vi "sych2SQL.vi"(11 "Data\\":path=path "\\\\192.168.1.45\\du lieu kho/data") -> ()   [LabVIEW 2015]
uses:
  <vilib>/addons/database/Connection.llb/Conn ObjectReference.ctl
  <vilib>/Utility/miscctls.llb/LVRowAndColumnUnsignedTypeDef.ctl
  <vilib>/addons/database/Connection.llb/DB Tools Open Connec (String).vi
  <vilib>/addons/database/Connection.llb/Conn Execute.vi
  <vilib>/addons/database/Recordset.llb/Rec Destroy - Connection.vi
  <vilib>/addons/database/NI_Database_API.lvlib
panel:
  out "error out 9":errorcluster
  out "Numeric 2":i32
  out "error out 8":errorcluster
  out "error out 3":errorcluster
  out "Array":errorcluster[](array[cluster])
  in  "connection reference 3":T1
  in  "connection reference 2":T1
  out "Numeric":i32
  out "error out 7":errorcluster
  out "error out 6":errorcluster
  out "error out 5":errorcluster
  out "error out 4":errorcluster
  out "error out 2":errorcluster
  out "error out":errorcluster
  in  "Lot Size":dbl
  out "Table 2":string[][](table)
  in  "Amount (F4)":dbl caption="(F4)"
  in  "Item Code (F3)":string
  out "ECODE":string
  in  "Input Date":timestamp format="%<%d/%m/%Y>T"
  out "Input No.":string
  in  "Product":string(combo)
  in  "Quantity":dbl
  in  "Location":string
  in  "Maker":string(combo)
  in  "Lot Maker":string
  in  "Maker Code":string
  in  "Unit 2":string
  in  "AUTO_PRINT":bool caption="AUTO"
  in  "connection reference":T1
  out "password":cluster{"ID":string, "Password":string}[](array[cluster])
  in  "Next Button 2":bool
  in  "Find":string
  out "Find Array":i32[](array[numeric])
  in  "output cluster 2":cluster{"ID":string, "Password":string}
  out "Worker Code":string
  out "record(s) 3":T2(array[cluster])
  in  "element 3":T3
  in  "Ring":u16(ring) items=["INVOICE", "LINE"]
  in  "element":T3
  out "record(s)":T2(array[cluster])
  in  "End":bool
  out "Item code":string[](array[string])
  out "Item data":T4(array[cluster])
  out "Initial":i32
  out "Output":i32
  out "Input":i32
  in  "Initial Date":string
  in  "Item type":T5
  in  "DATE":string
  in  "Invoice Date":string
  in  "Exit":bool
  in  "output array":string[][](array[string])=[["", "", "", "", "", "", "", ""]]
  in  "PRODUCT":string
  in  "input array":string[][](array[string])=[["", "", "", "", "", "", "", ""]]
  in  "Check":bool
  in  "Table":string[][](table)=[["", "", "", "", "", "", "", ""], ["", "", "", "", "", "", "", ""], ["", "", "", "", "", "", "", ""], ["", "", "", "", "", "", "", ""], ["", "", "", "", "", "", "", ""], ["", "", "", "", "", "", "", ""]]
  # "CHECK STOCK"
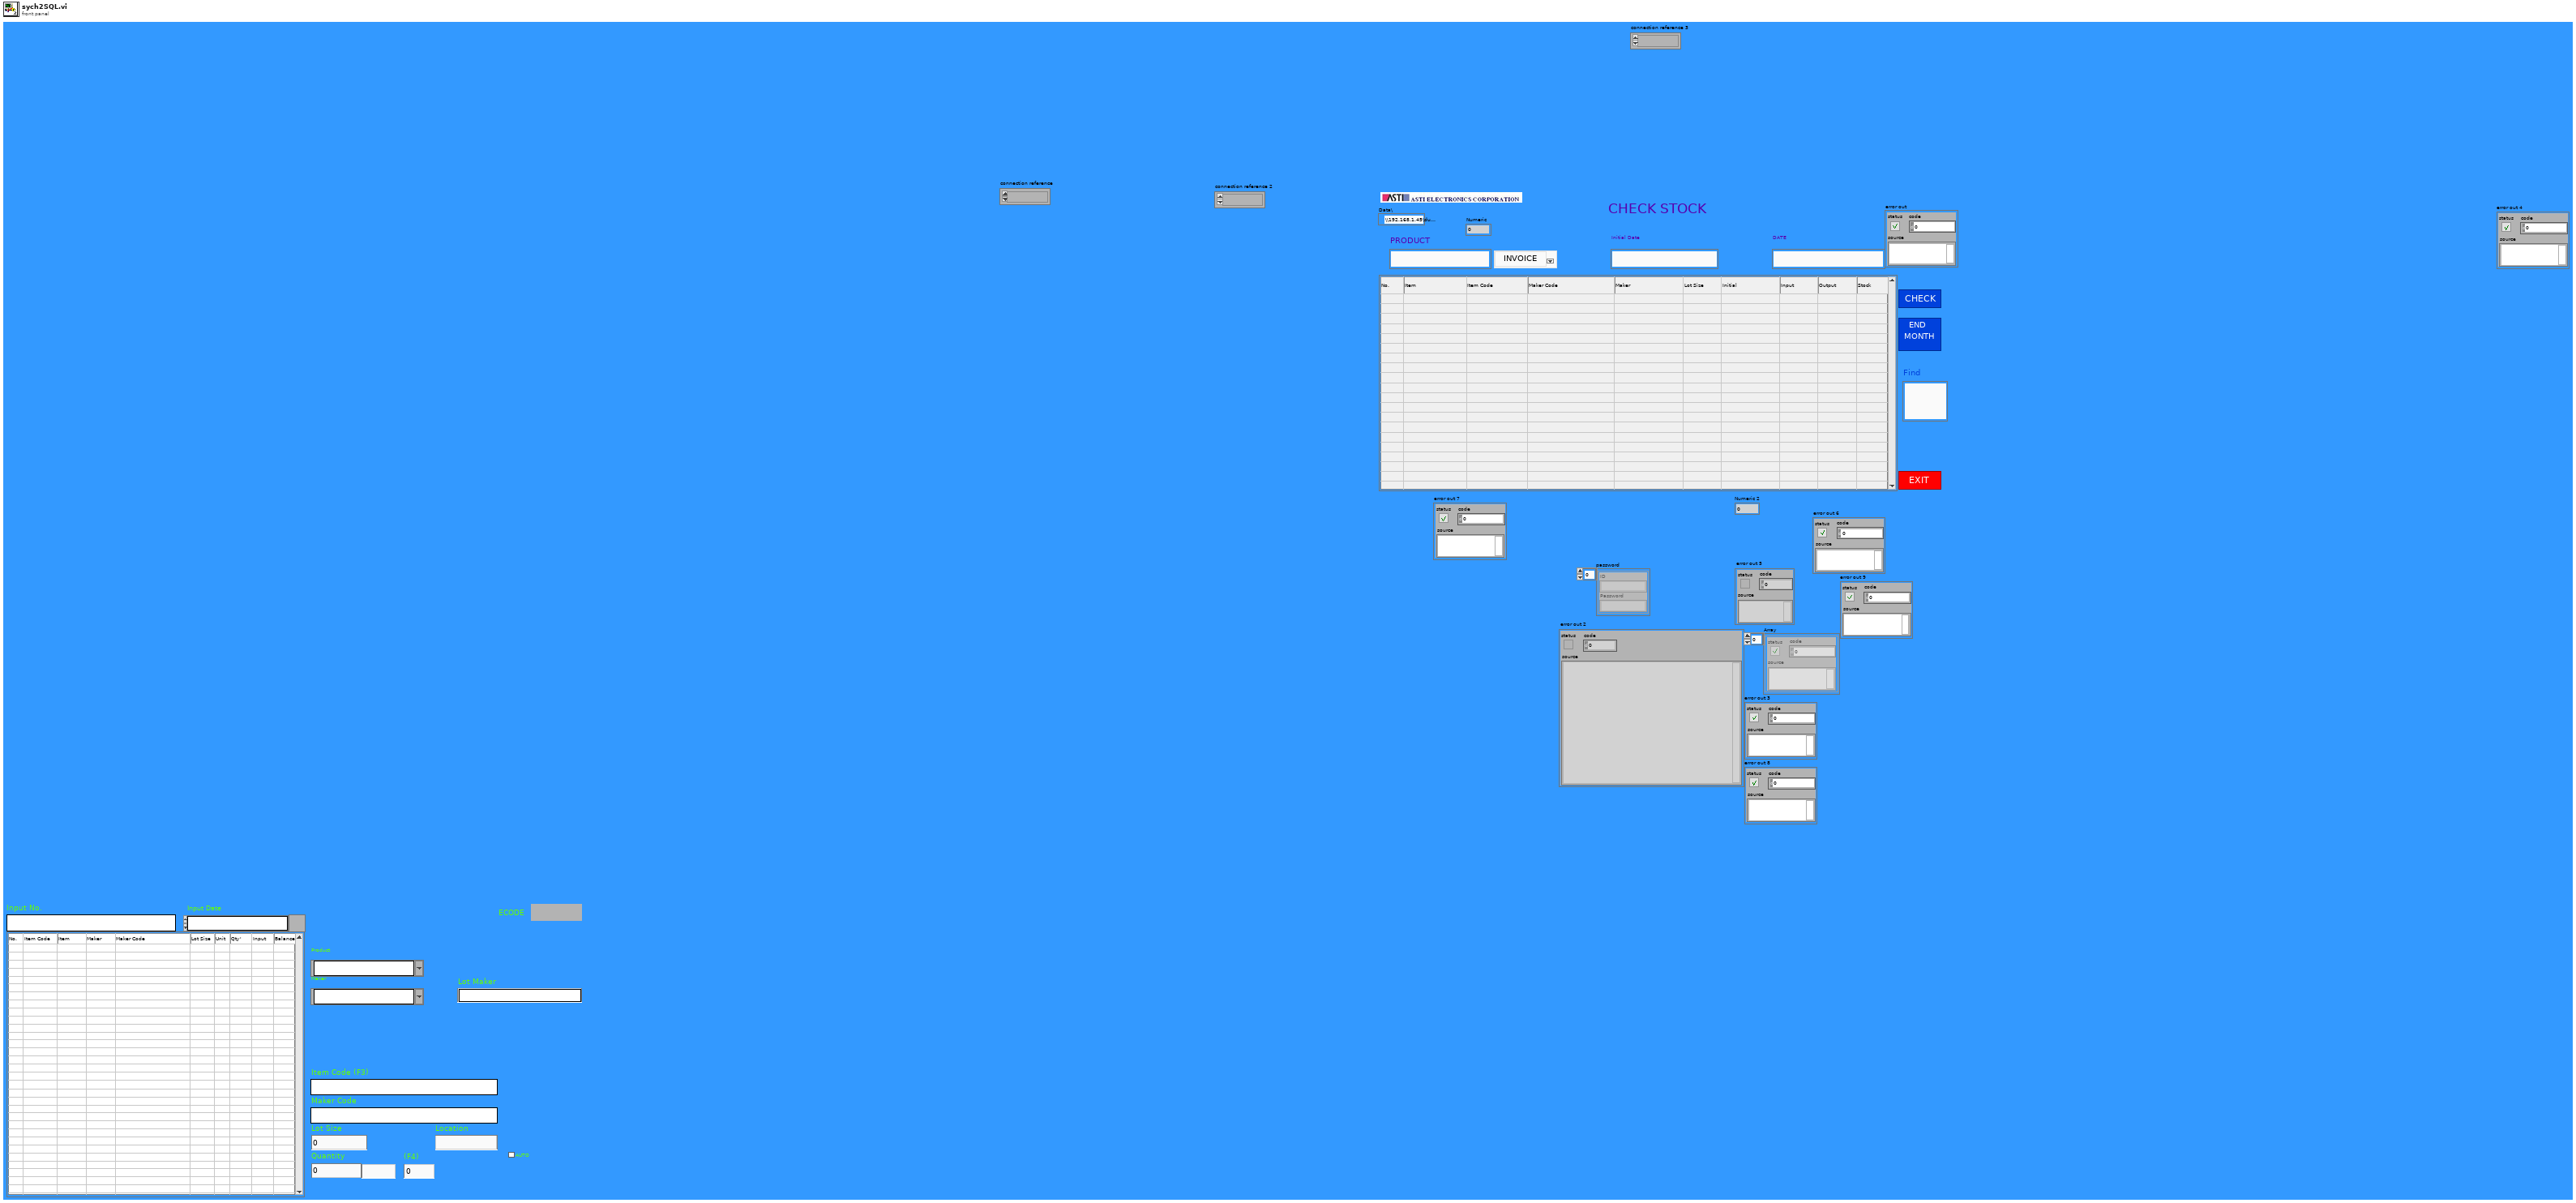
[diagram p1: front panel]
types:
  T1 = typedef "NI_Database_API.lvlib/Conn ObjectReference.ctl" = refnum<k1>
  T2 = cluster{"Item Code":string, "Initial":string, "End":string}[]
  T3 = cluster{"Item Code":string, "Initial":string, "End":string}
  T4 = cluster{"Maker Code":string, "Item Code":string, "Product":string, "Item":string, "Maker":string, "Lot Size":string, "Unit":string, "Tare":string, "Sample":string}[]
  T5 = cluster{"Maker Code":string, "Item Code":string, "Product":string, "Item":string, "Maker":string, "Lot Size":string, "Unit":string, "Tare":string, "Sample":string}
  T6 = enum8{"Enabled", "Disabled", "Disabled and Grayed Out"}
  T7 = cluster{"Product":string, "Item":string, "Item Code":string, "Maker Code":string, "Maker":string, "Lot Size":string, "Initial":i32, "Input":i32, "Output":i32, "End":i32}
  T8 = enum16{"open", "replace", "create", "open or create", "replace or create", "replace or create with confirmation"}
  T9 = cluster{"Inv Date":string, "Invoice":string, "Output Date":string, "Output No.":string, "Item Code":string, "Input":string, "Worker Code":string, "Dest":string}[]
  T10 = cluster{"Inv Date":string, "Invoice":string, "Output Date":string, "Output No.":string, "Item Code":string, "Input":string, "Worker Code":string, "Dest":string}
  T11 = typedef "LVRowAndColumnUnsignedTypeDef.ctl" = cluster{"Row":u32, "Column":u32}
  T12 = cluster{"ITEM_CODE":string, "INVOICE_NO":string, "INVOICE_DATE":timestamp, "LOT_MAKER":string, "QUANTITY":dbl, "INVOICE_ECODE":string, "INPUT_NO":string, "INPUT_DATE":timestamp, "INPUT_ECODE":string, "LINEBACK_NO":string, "LINEBACK_DATE":timestamp, "LINEBACK_ECODE":string, "OUTPUT_NO":string, "OUTPUT_DATE":timestamp, "OUTPUT_ECODE":string, "DESTINATION":string}
  T13 = typedef "NI_Database_API.lvlib/Rec ObjectReference.ctl" = refnum<k1>
  T14 = cluster{timestamp, "Output No.":string, "Worker Code":string}
  T15 = cluster{"Item Code":string, "Initial":string, "Stock":string}
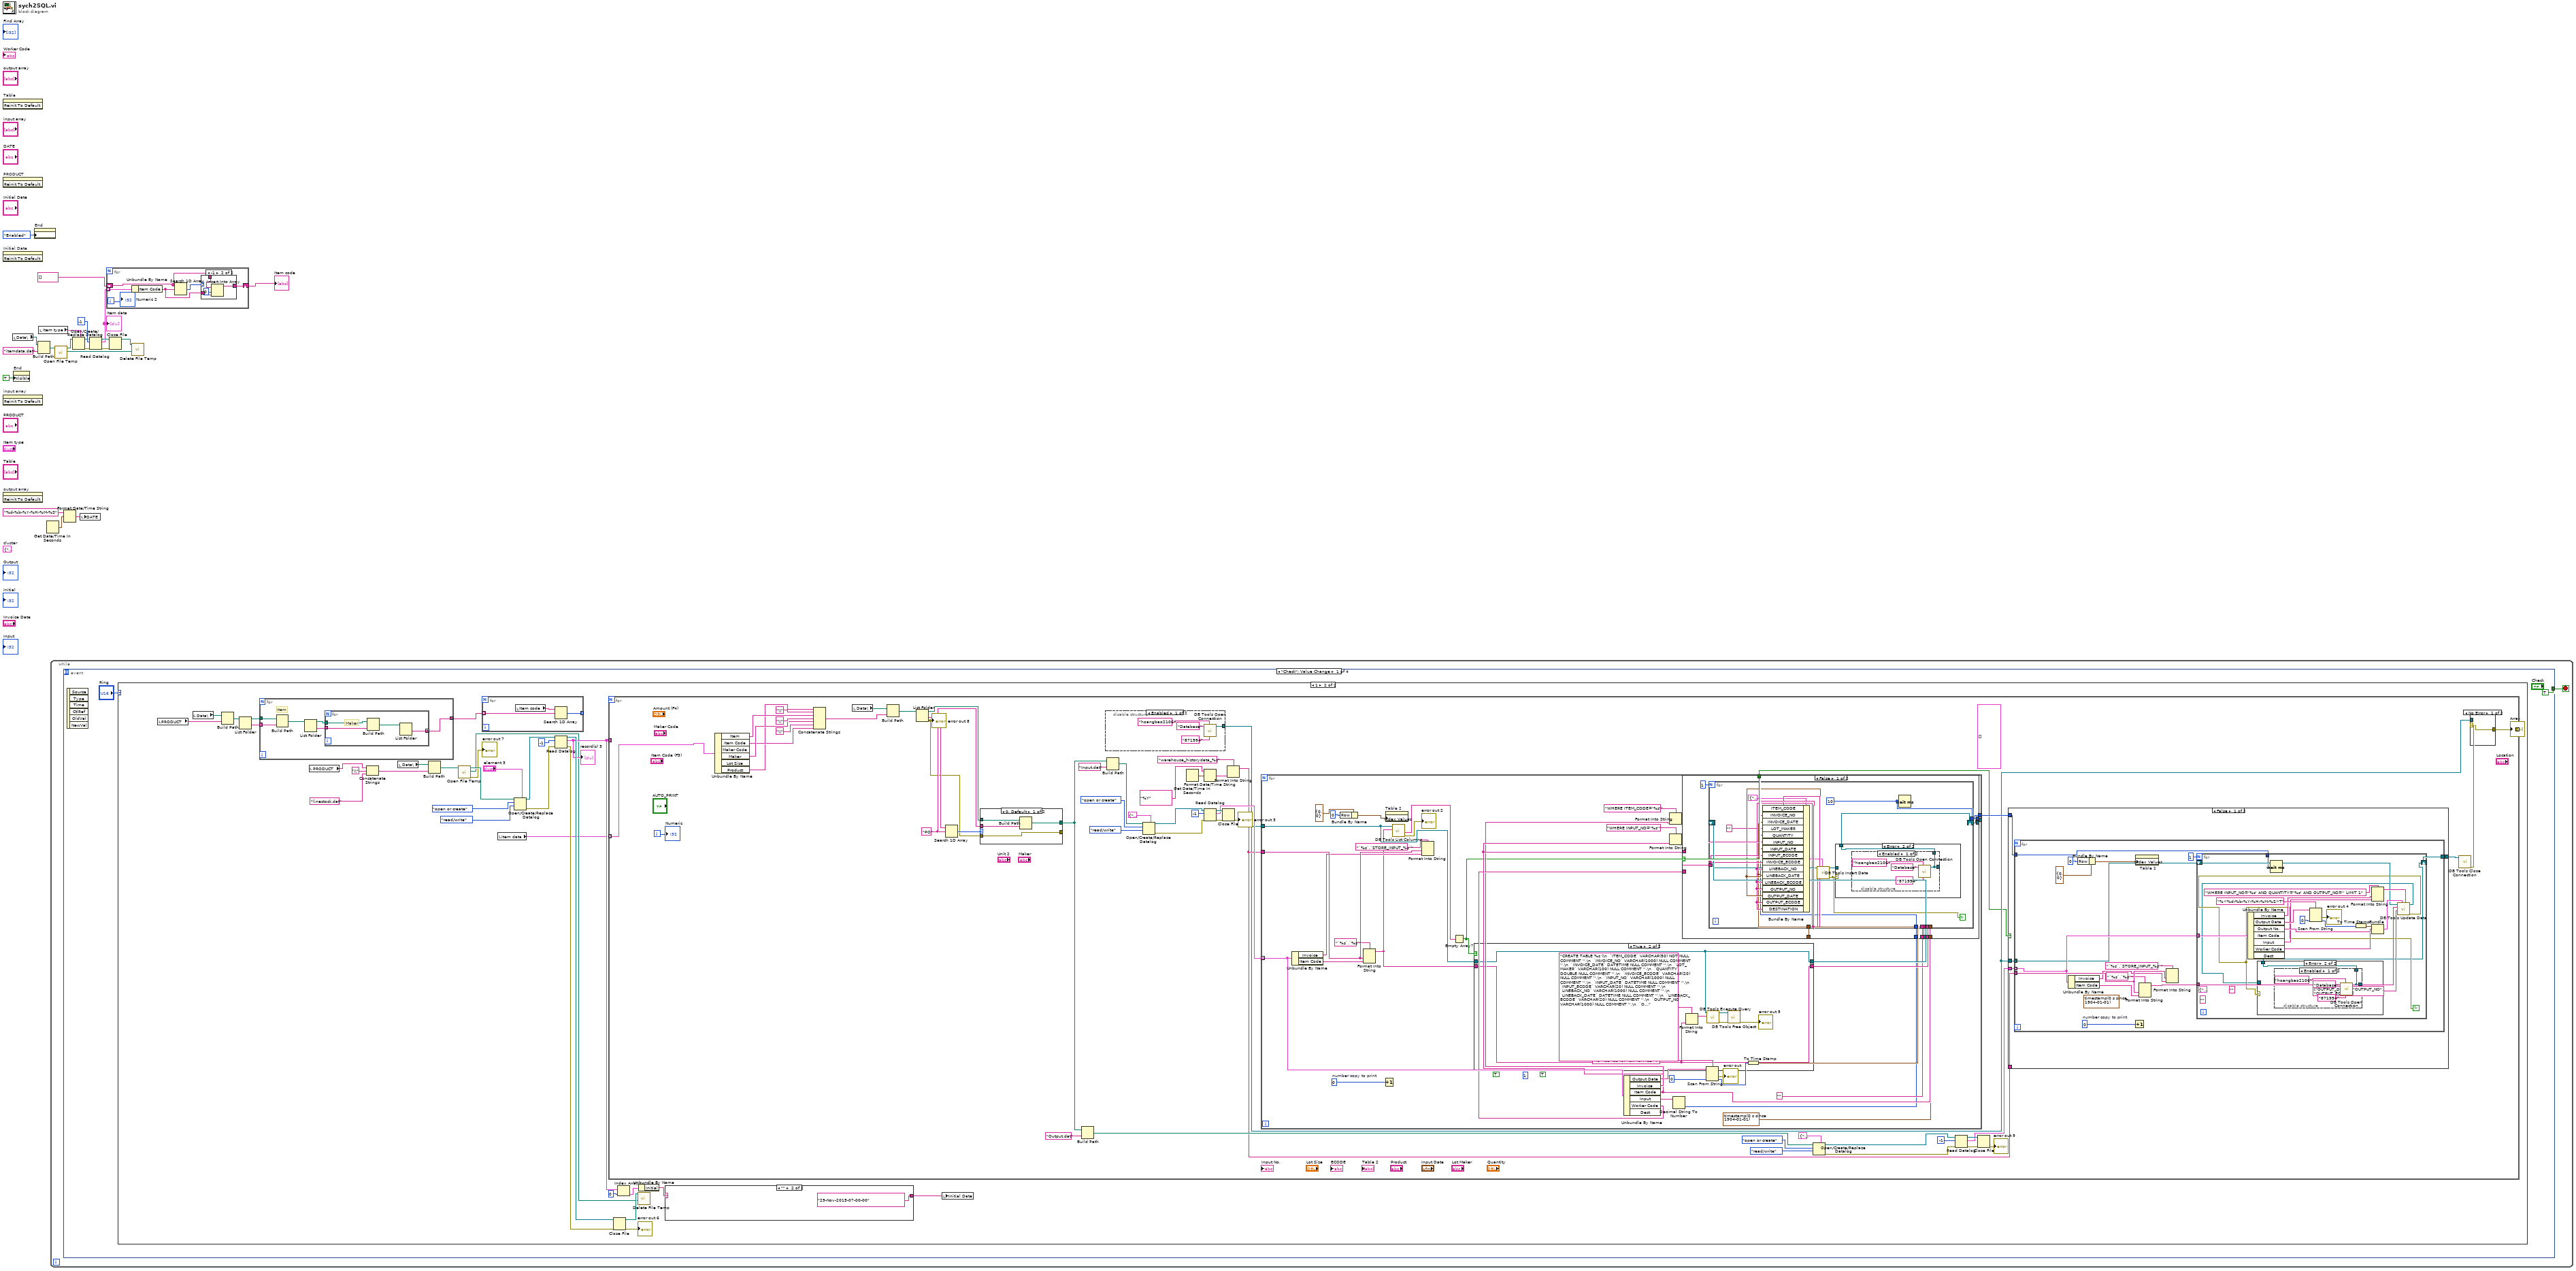
[diagram p0: block diagram]
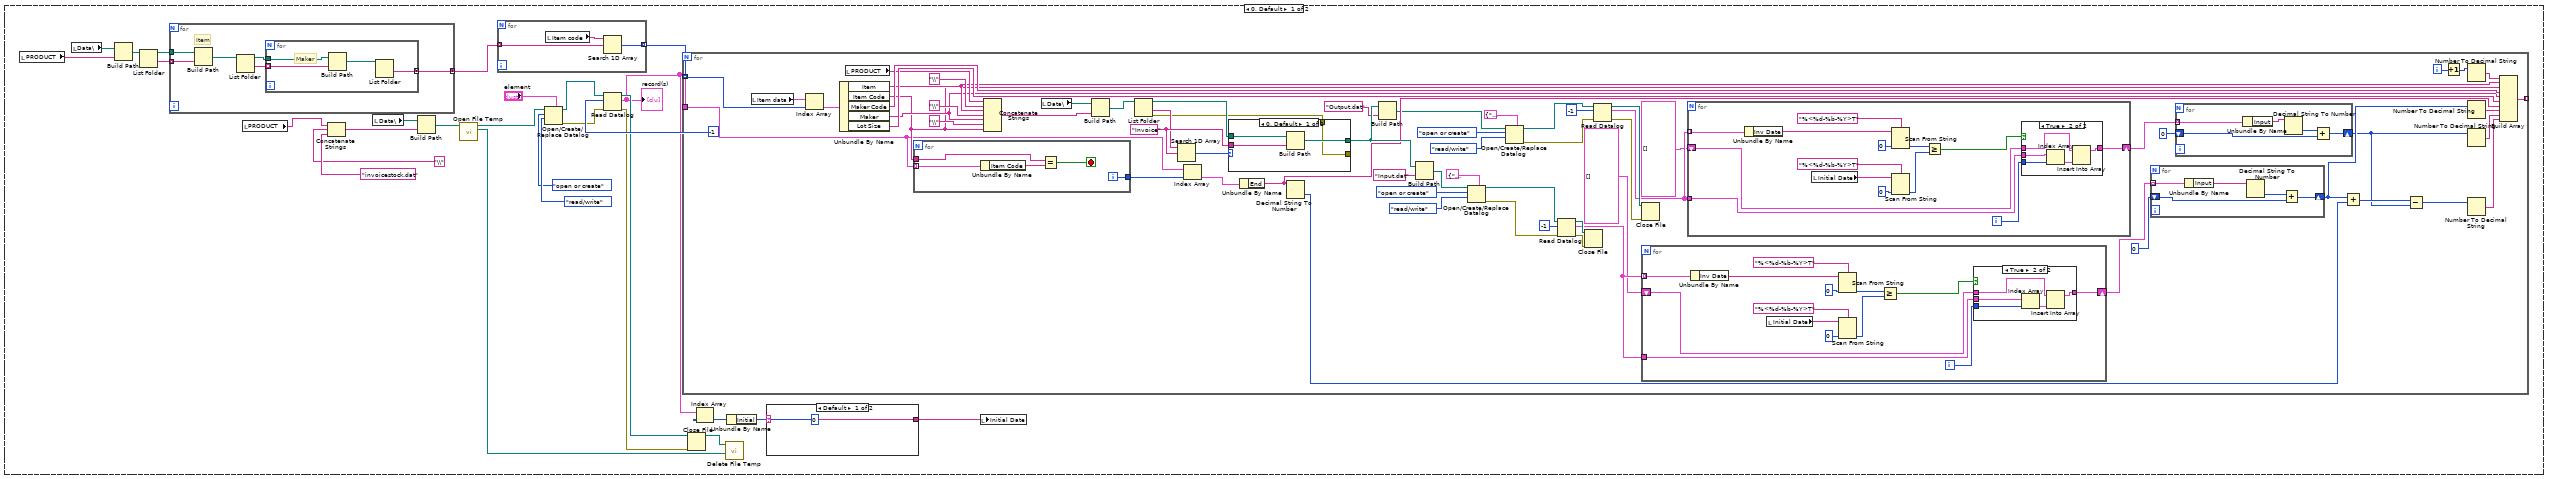
[diagram p2: hidden frame]
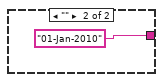
[diagram p3: hidden frame]
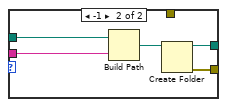
[diagram p6: hidden frame]
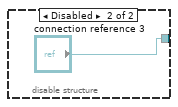
[diagram p9: hidden frame]
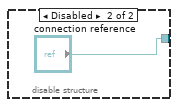
[diagram p11: hidden frame]
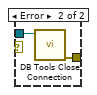
[diagram p12: hidden frame]
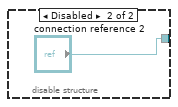
[diagram p14: hidden frame]
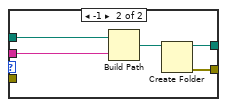
[diagram p17: hidden frame]
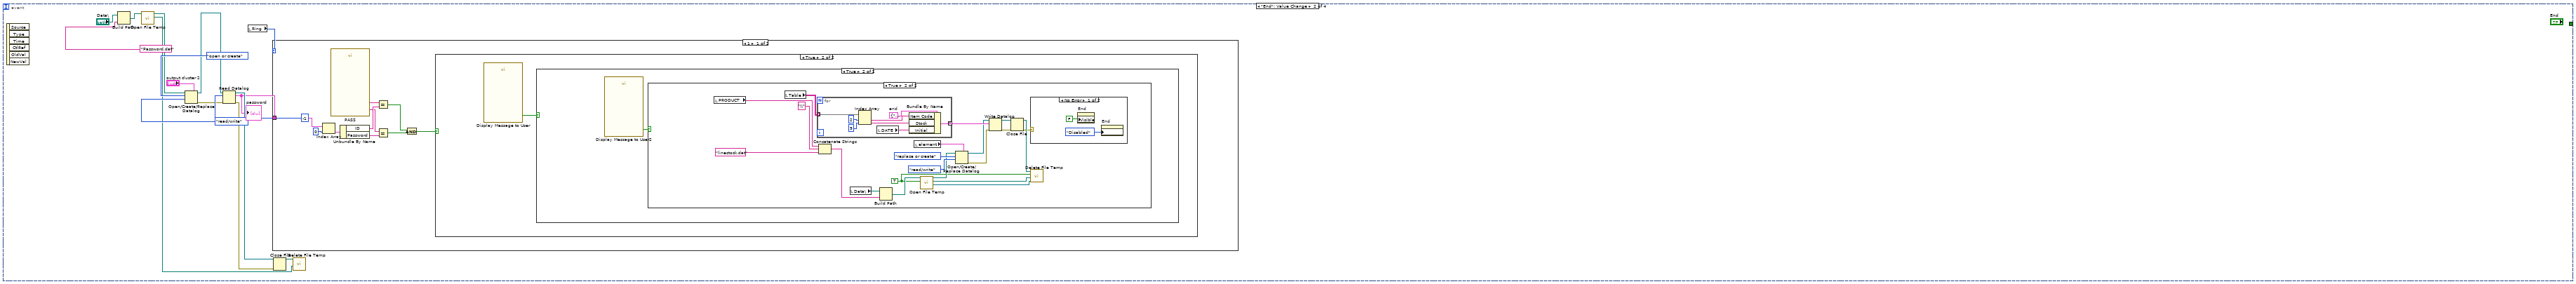
[diagram p18: hidden frame]
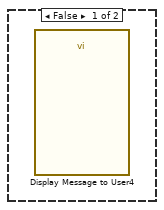
[diagram p19: hidden frame]
diagram:
  (unwired) T7 {"Product"="", "Item"="", "Item Code"="", "Maker Code"="", "Maker"="", "Lot Size"="", "Initial"=0, "Input"=0, "Output"=0, "End"=0}  # cluster
  n1 = invoke on="Table" class="Tbl (strict)" method="Reinit To Default"() -> ()  [unwired: 3 in, 3 out]
  n2 = invoke on="PRODUCT" class="Str" method="Reinit To Default"() -> ()  [unwired: 3 in, 3 out]
  n3 = invoke on="Initial Date" class="Str" method="Reinit To Default"() -> ()  [unwired: 3 in, 3 out]
  n4 = invoke on="input array" class="Arr (strict)" method="Reinit To Default"() -> ()  [unwired: 3 in, 3 out]
  n5 = invoke on="output array" class="Arr (strict)" method="Reinit To Default"() -> ()  [unwired: 3 in, 3 out]
  n6 = local read "Data\\"() -> (w14:path)
  n7 = property on="End" class="Bool"("Visible"=TRUE) -> ()  [unwired: 2 in, 2 out]
  n8 = property on="End" class="Bool"("DisabledEnum"=T6."Enabled" ("Disabled")) -> ()  [unwired: 2 in, 2 out]
  n9 = Build Path(base path=w14, name or relative path="itemdata.dat") -> (appended path=w8:path)
  n10 = local read "Item type"() -> (w16:T5)
  n11 = Get Date/Time In Seconds() -> (seconds since 1Jan1904=w20:timestamp)
  n12 = while {
    stop <- w21 stop-if-true
    n13 = event shown="[0] \"Check\": Value Change" {
      selector: _ -> [_ _ _ _]
      dyn-events: _ -> [_ _ _ _]
      timeout: _ -> [_ _ _ _]
      tunnel: [TRUE ("Exit") _ _ "Exit"] -> w21
      event "Check": Value Change {
        n14 = event-data() -> ()  [unwired: 1 in, 6 out]
        n15 = case shown="1" "Ring" {
          frame 0, Default {
            n16 = local read "PRODUCT"() -> (w51:string)
            n17 = local read "Data\\"() -> (w52:path)
            n18 = Build Path(base path=w52, name or relative path=w51) -> (appended path=w49:path)
            n19 = List Folder(path=w49) -> (path out=w48:path, folder names=w50:string[])  [unwired: 3 in, 2 out]
            n20 = for {
              tunnel: w50 -> [w191] mode=indexing
              tunnel: w48 -> [w192]
              tunnel: [w187] -> w47 mode=concatenating
              # "Item"
              n21 = Build Path(base path=w192, name or relative path=w191) -> (appended path=w189:path)
              n22 = List Folder(path=w189) -> (path out=w188:path, folder names=w190:string[])  [unwired: 3 in, 2 out]
              n23 = for {
                tunnel: w190 -> [w195] mode=indexing
                tunnel: w188 -> [w196]
                tunnel: [w194] -> w187 mode=concatenating
                # "Maker"
                n24 = Build Path(base path=w196, name or relative path=w195) -> (appended path=w193:path)
                n25 = List Folder(path=w193) -> (folder names=w194:string[])  [unwired: 3 in, 3 out]
              }
            }
            n26 = local read "PRODUCT"() -> (w44:string)
            n27 = Concatenate Strings(w44, "\\" ("string"), "invoicestock.dat" ("name or relative path")) -> (w45:string)
            n28 = local read "Data\\"() -> (w33:path)
            n29 = Build Path(base path=w33, name or relative path=w45) -> (appended path=w27:path)
            n30 = call "Open File Temp.vi"("Path file"=w27) -> ("Source Path"=w24:path, "Temp path"=w26:path)  [unwired: 7 in, 2 out]
            n31 = for {
              tunnel: w47 -> [w185] mode=indexing
              tunnel: [w184] -> w46 mode=indexing
              n32 = local read "Item code"() -> (w186:string[])
              n33 = Search 1D Array(1D array=w186, element=w185) -> (index of element=w184:i32)  [unwired: 1 in]
            }
            n34 = Open/Create/Replace Datalog(5:"element", 9:enum16{"read/write", "read-only", "write-only"}."read/write" ("access (0:read/write)"), 10:T8."open or create" ("operation (0:open)"), 11:w26) -> (0:w35:errorcluster, 3:w34:refnum<k1>)  [unwired: 2 in, 1 out]
            n35 = Read Datalog(4:w35, 6:-1 ("count (1)"), 7:w34) -> (0:w37:errorcluster, 2:w28:T2, 3:w36:refnum<k1>)
            "record(s)" <- w28
            n36 = for {
              tunnel: w46 -> [w118] mode=indexing
              tunnel: [w114] -> _ mode=indexing
              tunnel: w28 -> [w71]
              i -> [w113]
              w102 = "Invoice" ("string")
              n37 = local read "Item data"() -> (w119:T4)
              n38 = Index Array(array=w119, index=w118) -> (element=w117:T5)
              n39 = Unbundle By Name(w117) -> ("Item"=w92:string, "Item Code"=w72:string, "Maker Code"=w116:string, "Maker"=w91:string, "Lot Size"=w115:string)
              n40 = local read "PRODUCT"() -> (w108:string)
              n41 = for {
                tunnel: w71 -> [w124] mode=indexing
                tunnel: w72 -> [w123]
                tunnel: [w120] -> w70
                i -> [w120]
                stop <- w121 stop-if-true
                n42 = Unbundle By Name(w124) -> ("Item Code"=w122:string)
                n43 = Equal?(x=w123, y=w122) -> (x = y?=w121:bool)
              }
              n44 = Concatenate Strings(w108, "\\" ("string"), w92, "\\" ("string"), w91, "\\" ("string"), w72) -> (w105:string)
              n45 = local read "Data\\"() -> (w106:path)
              n46 = Build Path(base path=w106, name or relative path=w105) -> (appended path=w110:path)
              n47 = List Folder(path=w110) -> (path out=w93:path, folder names=w94:string[], error out=w55:errorcluster)  [unwired: 3 in, 1 out]
              n48 = Search 1D Array(1D array=w94, element=w102) -> (index of element=w104:i32)  [unwired: 1 in]
              n49 = Index Array(array=w71, index=w70) -> (element=w69:T3)
              n50 = case shown="0, Default" w104 {
                tunnel: w93 -> [w178 w183]
                tunnel: [w177 w181] -> w80
                tunnel: w102 -> [w176 w180]
                tunnel: [w175 w179] -> _
                tunnel: w55 -> [w175 _]
                frame 0, Default {
                  n51 = Build Path(base path=w178, name or relative path=w176) -> (appended path=w177:path)
                }
                frame -1 {
                  n52 = Build Path(base path=w183, name or relative path=w180) -> (appended path=w182:path)
                  n53 = Create Folder(path (use dialog)=w182) -> (created path=w181:path, error out=w179:errorcluster)  [unwired: 2 in, 1 out]
                }
              }
              n54 = Unbundle By Name(w69) -> ("End"=w68:string)
              n55 = Decimal String To Number(string=w68) -> (number=w67:i32)  [unwired: 2 in, 1 out]
              n56 = Build Path(base path=w80, name or relative path="Output.dat" ("string")) -> (appended path=w61:path)
              n57 = Build Path(base path=w80, name or relative path="Input.dat" ("string")) -> (appended path=w62:path)
              n58 = Open/Create/Replace Datalog(5:T10 {"Inv Date"="", "Invoice"="", "Output Date"="", "Output No."="", "Item Code"="", "Input"="", "Worker Code"="", "Dest"=""}, 9:enum16{"read/write", "read-only", "write-only"}."read/write" ("access (0:read/write)"), 10:T8."open or create" ("operation (0:open)"), 11:w62) -> (0:w98:errorcluster, 3:w97:refnum<k1>)  [unwired: 2 in, 1 out]
              n59 = Open/Create/Replace Datalog(5:T10 {"Inv Date"="", "Invoice"="", "Output Date"="", "Output No."="", "Item Code"="", "Input"="", "Worker Code"="", "Dest"=""}, 9:enum16{"read/write", "read-only", "write-only"}."read/write" ("access (0:read/write)"), 10:T8."open or create" ("operation (0:open)"), 11:w61) -> (0:w83:errorcluster, 3:w84:refnum<k1>)  [unwired: 2 in, 1 out]
              n60 = Read Datalog(4:w98, 6:-1 ("count (1)"), 7:w97) -> (0:w89:errorcluster, 2:w60:T9, 3:w90:refnum<k1>)
              n61 = Close File(refnum=w90, error in=w89) -> ()  [unwired: 2 out]
              n62 = Read Datalog(4:w83, 6:-1 ("count (1)"), 7:w84) -> (0:w88:errorcluster, 2:w73:T9, 3:w87:refnum<k1>)
              n63 = Close File(refnum=w87, error in=w88) -> ()  [unwired: 2 out]
              n64 = for {
                tunnel: w60 -> [w145] mode=indexing
                tunnel: w60 -> [w150]
                shift-right: [w148] -> w58
                shift-left: T9 [] ("record(s)") -> [w149]
                i -> [w146]
                n65 = Unbundle By Name(w145) -> ("Inv Date"=w156:string)
                n66 = local read "Initial Date"() -> (w153:string)
                n67 = Scan From String(format string="%<%d-%b-%Y>T", input string=w156, default 1=i64 0) -> (output 1=w152:i64)  [unwired: 2 in, 3 out]
                n68 = Scan From String(format string="%<%d-%b-%Y>T", input string=w153, default 1=i64 0) -> (output 1=w151:i64)  [unwired: 2 in, 3 out]
                n69 = Greater Or Equal?(x=w152, y=w151) -> (x >= y?=w147:bool)
                n70 = case shown="True" w147 {
                  tunnel: w150 -> [_ w164]
                  tunnel: [w159 w161] -> w148
                  tunnel: w146 -> [_ w163]
                  tunnel: w149 -> [w159 w162]
                  frame False {
                  }
                  frame True {
                    n71 = Index Array(array=w164, index=w163) -> (element=w160:T10)
                    n72 = Insert Into Array(array=w162, new element=w160) -> (w161:T9)  [unwired: 1 in]
                  }
                }
              }
              n73 = for {
                tunnel: w73 -> [w128]
                tunnel: w73 -> [w126] mode=indexing
                shift-right: [w127] -> w56
                shift-left: T9 [] ("record(s)") -> [w129]
                i -> [w125]
                n74 = Unbundle By Name(w126) -> ("Inv Date"=w136:string)
                n75 = local read "Initial Date"() -> (w133:string)
                n76 = Scan From String(format string="%<%d-%b-%Y>T", input string=w136, default 1=i64 0) -> (output 1=w132:i64)  [unwired: 2 in, 3 out]
                n77 = Scan From String(format string="%<%d-%b-%Y>T", input string=w133, default 1=i64 0) -> (output 1=w131:i64)  [unwired: 2 in, 3 out]
                n78 = Greater Or Equal?(x=w132, y=w131) -> (x >= y?=w130:bool)
                n79 = case shown="True" w130 {
                  tunnel: w128 -> [_ w144]
                  tunnel: [w139 w142] -> w127
                  tunnel: w129 -> [w139 w143]
                  tunnel: w125 -> [_ w140]
                  frame False {
                  }
                  frame True {
                    n80 = Index Array(array=w144, index=w140) -> (element=w141:T10)
                    n81 = Insert Into Array(array=w143, new element=w141) -> (w142:T9)  [unwired: 1 in]
                  }
                }
              }
              n82 = for {
                tunnel: w58 -> [w174] mode=indexing
                shift-right: [w171] -> w66
                shift-left: 0 -> [w170]
                n83 = Unbundle By Name(w174) -> ("Input"=w173:string)
                n84 = Decimal String To Number(string=w173) -> (number=w172:i32)  [unwired: 2 in, 1 out]
                n85 = Add(x=w172, y=w170) -> (x+y=w171:i32)
              }
              n86 = for {
                tunnel: w56 -> [w169] mode=indexing
                shift-right: [w166] -> w64
                shift-left: 0 -> [w165]
                n87 = Unbundle By Name(w169) -> ("Input"=w168:string)
                n88 = Decimal String To Number(string=w168) -> (number=w167:i32)  [unwired: 2 in, 1 out]
                n89 = Add(x=w167, y=w165) -> (x+y=w166:i32)
              }
              n90 = Add(x=w66, y=w67) -> (x+y=w65:i32)
              n91 = Subtract(x=w65, y=w64) -> (x-y=w63:i32)
              n92 = Increment(x=w113) -> (x+1=w112:i32)
              n93 = Number To Decimal String(number=w112) -> (decimal integer string=w111:string)  [unwired: 1 in]
              n94 = Number To Decimal String(number=w66) -> (decimal integer string=w76:string)  [unwired: 1 in]
              n95 = Number To Decimal String(number=w64) -> (decimal integer string=w75:string)  [unwired: 1 in]
              n96 = Number To Decimal String(number=w63) -> (decimal integer string=w74:string)  [unwired: 1 in]
              n97 = Build Array(w111, w92, w72, w116, w91, w115, w68, w76, w75, w74) -> (w114:string[])
            }
            n98 = Close File(refnum=w36, error in=w37) -> (path=w25:path)  [unwired: 1 out]
            n99 = Index Array(array=w28, index=0) -> (element=w31:T3)
            n100 = call "Delete File Temp.vi"("Source Path"=w24, "Temp path"=w25) -> ()  [unwired: 8 in, 2 out]
            n101 = Unbundle By Name(w31) -> ("Initial"=w30:string)
            n102 = case shown="Default" w30 {
              selector: w30 -> [w53 _]
              tunnel: [w53 "01-Jan-2010"] -> w29
              frame Default {
              }
              frame "" {
              }
            }
            n103 = local write "Initial Date"(w29) -> ()
          }
          frame 1 {
            n104 = local read "PRODUCT"() -> (w227:string)
            n105 = local read "Data\\"() -> (w228:path)
            n106 = Build Path(base path=w228, name or relative path=w227) -> (appended path=w225:path)
            n107 = List Folder(path=w225) -> (path out=w224:path, folder names=w226:string[])  [unwired: 3 in, 2 out]
            n108 = for {
              tunnel: w226 -> [w436] mode=indexing
              tunnel: w224 -> [w437]
              tunnel: [w432] -> w223 mode=concatenating
              # "Item"
              n109 = Build Path(base path=w437, name or relative path=w436) -> (appended path=w434:path)
              n110 = List Folder(path=w434) -> (path out=w433:path, folder names=w435:string[])  [unwired: 3 in, 2 out]
              n111 = for {
                tunnel: w435 -> [w440] mode=indexing
                tunnel: w433 -> [w441]
                tunnel: [w439] -> w432 mode=concatenating
                # "Maker"
                n112 = Build Path(base path=w441, name or relative path=w440) -> (appended path=w438:path)
                n113 = List Folder(path=w438) -> (folder names=w439:string[])  [unwired: 3 in, 3 out]
              }
            }
            n114 = local read "PRODUCT"() -> (w221:string)
            n115 = Concatenate Strings(w221, "\\" ("string"), "linestock.dat" ("name or relative path")) -> (w222:string)
            n116 = local read "Data\\"() -> (w210:path)
            n117 = Build Path(base path=w210, name or relative path=w222) -> (appended path=w204:path)
            n118 = call "Open File Temp.vi"("Path file"=w204) -> ("error out"=→"error out 7":errorcluster, "Source Path"=w201:path, "Temp path"=w203:path)  [unwired: 7 in, 1 out]
            n119 = for {
              tunnel: w223 -> [w430] mode=indexing
              tunnel: [w429] -> _ mode=indexing
              n120 = local read "Item code"() -> (w431:string[])
              n121 = Search 1D Array(1D array=w431, element=w430) -> (index of element=w429:i32)  [unwired: 1 in]
            }
            n122 = local read "Item data"() -> (w197:T4)
            n123 = Open/Create/Replace Datalog(5:"element 3", 9:enum16{"read/write", "read-only", "write-only"}."read/write" ("access (0:read/write)"), 10:T8."open or create" ("operation (0:open)"), 11:w203) -> (0:w212:errorcluster, 3:w211:refnum<k1>)  [unwired: 2 in, 1 out]
            n124 = Read Datalog(4:w212, 6:-1 ("count (1)"), 7:w211) -> (0:w214:errorcluster, 2:w205:T2, 3:w213:refnum<k1>)
            "record(s) 3" <- w205
            n125 = for {
              tunnel: w205 -> [_]
              tunnel: [w236] -> w198 mode=indexing
              tunnel: w197 -> [w234] mode=indexing
              i -> [w238]
              (unwired) T9 [] ("record(s)")
              w276 = "PO" ("string")
              n126 = Unbundle By Name(w234) -> ("Item"=w266:string, "Item Code"=w253:string, "Maker"=w265:string, "Product"=w233:string)  [unwired: 2 out]
              n127 = Concatenate Strings(w233, "\\" ("string"), w266, "\\" ("string"), w265, "\\" ("string"), w253) -> (w279:string)
              n128 = local read "Data\\"() -> (w280:path)
              n129 = Build Path(base path=w280, name or relative path=w279) -> (appended path=w283:path)
              n130 = List Folder(path=w283) -> (path out=w267:path, folder names=w268:string[], error out=w231:errorcluster)  [unwired: 3 in, 1 out]
              "error out 8" <- w231
              n131 = Search 1D Array(1D array=w268, element=w276) -> (index of element=w278:i32)  [unwired: 1 in]
              n132 = case shown="0, Default" w278 {
                tunnel: w267 -> [w423 w428]
                tunnel: [w422 w426] -> w250
                tunnel: w276 -> [w421 w425]
                tunnel: [w420 w424] -> _
                tunnel: w231 -> [w420 _]
                frame 0, Default {
                  n133 = Build Path(base path=w423, name or relative path=w421) -> (appended path=w422:path)
                }
                frame -1 {
                  n134 = Build Path(base path=w428, name or relative path=w425) -> (appended path=w427:path)
                  n135 = Create Folder(path (use dialog)=w427) -> (created path=w426:path, error out=w424:errorcluster)  [unwired: 2 in, 1 out]
                }
              }
              n136 = Build Path(base path=w250, name or relative path="Output.dat" ("string")) -> (appended path=w251:path)
              n137 = disable-structure shown="Enabled" {
                disable-tunnel: [w333 "connection reference"] -> w239
                frame Enabled {
                  n138 = call-poly <vilib>:"DB Tools Open Connection.vi"("password"="871994" ("userID"), "userID"="hoangbao2106", "connection information"="Database" ("userID")) -> ("connection reference"=w333:T1)  [unwired: 5 in, 1 out]
                }
                frame Disabled {
                }
              }
              n139 = Build Path(base path=w250, name or relative path="Input.dat" ("string")) -> (appended path=w252:path)
              n140 = Open/Create/Replace Datalog(5:T10 {"Inv Date"="", "Invoice"="", "Output Date"="", "Output No."="", "Item Code"="", "Input"="", "Worker Code"="", "Dest"=""}, 9:enum16{"read/write", "read-only", "write-only"}."read/write" ("access (0:read/write)"), 10:T8."open or create" ("operation (0:open)"), 11:w252) -> (0:w272:errorcluster, 3:w271:refnum<k1>)  [unwired: 2 in, 1 out]
              n141 = Get Date/Time In Seconds() -> (seconds since 1Jan1904=w247:timestamp)
              n142 = Format Date/Time String(time format string (%c)="%Y", seconds (now)=w247) -> (date/time string=w249:string)  [unwired: 1 in]
              n143 = Read Datalog(4:w272, 6:-1 ("count (1)"), 7:w271) -> (0:w263:errorcluster, 2:w245:T9, 3:w264:refnum<k1>)
              n144 = Close File(refnum=w264, error in=w263) -> (error out=→"error out 3":errorcluster)  [unwired: 1 out]
              n145 = Format Into String(format string="warehouse_historydata_%s" ("table"), w249) -> (resulting string=w244:string)  [unwired: 2 in, 1 out]
              n146 = for {
                tunnel: w239 -> [w369]
                tunnel: w244 -> [w374]
                tunnel: w245 -> [w370] mode=indexing
                tunnel: [w343] -> _
                tunnel: [w342] -> w240
                tunnel: [w341] -> w237
                (unwired) TRUE
                (unwired) 1
                w367 = 0  # number copy to print
                (unwired) TRUE
                n147 = Unbundle By Name(w370) -> ("Invoice"=w372:string, "Item Code"=w371:string)
                n148 = Bundle By Name(cluster=T11 {"Row"=0, "Column"=0} ("Index Values"), "Row"=0 ("index of element")) -> (w366:T11)
                n149 = Format Into String(format string="`%s`.`%s`", w374, w371) -> (resulting string=w356:string)  [unwired: 2 in, 1 out]
                n150 = Increment(x=w367) -> ()  [unwired: 1 out]
                n151 = property on="Table 2" class="Tbl (strict)"("Index Values"=w366) -> ()  [unwired: 2 in, 2 out]
                n152 = call <vilib>:"DB Tools List Columns.vi"("table"=w356, "connection reference"=w369) -> ("error out"=→"error out 2":errorcluster, "columns"=w357:string[])  [unwired: 2 in, 2 out]
                n153 = Format Into String(format string="`%s`.`STORE_INPUT_%s`", w374, w372) -> ()  [unwired: 2 in, 2 out]
                n154 = Empty Array?(array=w357) -> (empty?=w341:bool)
                n155 = case shown="True" w341 {
                  tunnel: w369 -> [w412 w413]
                  tunnel: w356 -> [w411 w415]
                  tunnel: [w411 w415] -> w354
                  tunnel: [w412 w413] -> w355
                  frame False {
                  }
                  frame True {
                    n156 = Format Into String(format string="CREATE TABLE %s (\n  `ITEM_CODE` VARCHAR(50) NOT NULL COMMENT '',\n  `INVOICE_NO` VARCHAR(1000) NULL COMMENT '',\n  `INVOICE_DATE` DATETIME NULL COMMENT '',\n  `LOT_MAKER` VARCHAR(100) NULL COMMENT '',\n  `QUANTITY` DOUBLE NULL COMMENT '',\n  `INVOICE_ECODE` VARCHAR(20) NULL COMMENT '',\n  `INPUT_NO` VARCHAR(1000) NULL COMMENT '',\n  `INPUT_DATE` DATETIME NULL COMMENT '',\n  `INPUT_ECODE` VARCHAR(20) NULL COMMENT '',\n  `LINEBACK_NO` VARCHAR(1000) NULL COMMENT '',\n  `LINEBACK_DATE` DATETIME NULL COMMENT '',\n  `LINEBACK_ECODE` VARCHAR(20) NULL COMMENT '',\n  `OUTPUT_NO` VARCHAR(1000) NULL COMMENT '',\n  `OUTPUT_DATE` DATETIME NULL COMMENT '',\n  `OUTPUT_ECODE` VARCHAR(20) NULL COMMENT '',\n  `DESTINATION` VARCHAR(1000) NULL COMMENT '');\n", w415) -> (resulting string=w416:string)  [unwired: 2 in, 1 out]
                    n157 = call-poly <vilib>:"DB Tools Execute Query.vi"("SQL query"=w416, "connection reference"=w413) -> ("error out"=w419:errorcluster, "recordset reference"=w418:T13)  [unwired: 6 in]
                    n158 = call-poly <vilib>:"DB Tools Free Object.vi"("error in (no error)"=w419, "recordset reference"=w418) -> ("error out"=→"error out 5":errorcluster)  [unwired: 8 in, 1 out]
                  }
                }
                n159 = Unbundle By Name(w370) -> ("Output Date"=w345:string, "Invoice"=w364:string, "Item Code"=w359:string, "Input"=w347:string, "Worker Code"=w363:string)  [unwired: 1 out]
                n160 = Format Into String(format string="WHERE ITEM_CODE='%s'" ("condition"), w359) -> ()  [unwired: 2 in, 2 out]
                n161 = Format Into String(format string="WHERE INPUT_NO='%s'" ("condition"), w364) -> ()  [unwired: 2 in, 2 out]
                n162 = Decimal String To Number(string=w347) -> (number=w348:i32)  [unwired: 2 in, 1 out]
                n163 = Scan From String(format string="%<%d-%b-%Y-%H-%M-%S>T", input string=w345, default 1=i64 0) -> (error out=→"error out":errorcluster, output 1=w360:i64)  [unwired: 2 in, 2 out]
                n164 = To Time Stamp(1:w360) -> (0:w349:timestamp)
                n165 = case shown="False" w341 {
                  tunnel: w364 -> [w386 _]
                  tunnel: w363 -> [w385 _]
                  tunnel: w359 -> [w384 _]
                  tunnel: w355 -> [w383 w410]
                  tunnel: w354 -> [w382 _]
                  tunnel: timestamp(0 s since 1904-01-01) ("OUTPUT_DATE") -> [w381 _]
                  tunnel: "" ("OUTPUT_NO") -> [w380 _]
                  tunnel: w349 -> [w379 _]
                  tunnel: w348 -> [w378 _]
                  tunnel: [w377 w410] -> w343
                  tunnel: [w376 _] -> w342
                  frame False {
                    n166 = for {
                      N: 1 -> [_]
                      tunnel: w386 -> [w402]
                      tunnel: w385 -> [w401]
                      tunnel: w384 -> [w400]
                      tunnel: w382 -> [w396]
                      tunnel: w381 -> [w395]
                      tunnel: w380 -> [w394]
                      tunnel: w379 -> [w393]
                      tunnel: w378 -> [w391]
                      tunnel: [w390] -> w376
                      shift-right: [w388] -> w377
                      shift-left: w383 -> [w398]
                      stop <- w387 continue-if-true
                      w390 = u32 10 ("milliseconds to wait")
                      n167 = Bundle By Name(cluster=T12 {"ITEM_CODE"="", "INVOICE_NO"="", "INVOICE_DATE"=timestamp(0 s since 1904-01-01), "LOT_MAKER"="", "QUANTITY"=0.0, "INVOICE_ECODE"="", "INPUT_NO"="", "INPUT_DATE"=timestamp(0 s since 1904-01-01), "INPUT_ECODE"="", "LINEBACK_NO"="", "LINEBACK_DATE"=timestamp(0 s since 1904-01-01), "LINEBACK_ECODE"="", "OUTPUT_NO"="", "OUTPUT_DATE"=timestamp(0 s since 1904-01-01), "OUTPUT_ECODE"="", "DESTINATION"=""}, "ITEM_CODE"=w400, "INVOICE_NO"=w402, "INVOICE_DATE"=w393, "LOT_MAKER"="", "QUANTITY"=w391, "INPUT_NO"=w402, "INPUT_DATE"=w393, "INPUT_ECODE"=w401, "INVOICE_ECODE"=w401, "LINEBACK_NO"=w394, "LINEBACK_DATE"=w395, "LINEBACK_ECODE"=w394, "OUTPUT_NO"=w394, "OUTPUT_DATE"=w395, "OUTPUT_ECODE"=w394, "DESTINATION"=w394) -> (w397:T12)
                      n168 = call <vilib>:"DB Tools Insert Data.vi"("data"=w397, "table"=w396, "connection reference"=w398) -> ("error out"=w387:errorcluster, "connection reference out"=w389:T1)  [unwired: 7 in]
                      n169 = case shown="Error" w387 {
                        tunnel: w389 -> [w403 _]
                        tunnel: [w403 w404] -> w388
                        frame No Error {
                        }
                        frame Error {
                          n170 = disable-structure shown="Enabled" {
                            disable-tunnel: [w405 "connection reference 2"] -> _
                            disable-tunnel: [w405 _] -> w404
                            frame Enabled {
                              n171 = call-poly <vilib>:"DB Tools Open Connection.vi"("password"="871994" ("userID"), "userID"="hoangbao2106", "connection information"="Database" ("userID")) -> ("connection reference"=w405:T1)  [unwired: 5 in, 1 out]
                            }
                            frame Disabled {
                            }
                          }
                        }
                      }
                      n172 = Wait (ms)(milliseconds to wait=w390) -> ()  [unwired: 1 out]
                    }
                  }
                  frame True {
                  }
                }
              }
              n173 = Open/Create/Replace Datalog(5:T10 {"Inv Date"="", "Invoice"="", "Output Date"="", "Output No."="", "Item Code"="", "Input"="", "Worker Code"="", "Dest"=""}, 9:enum16{"read/write", "read-only", "write-only"}."read/write" ("access (0:read/write)"), 10:T8."open or create" ("operation (0:open)"), 11:w251) -> (0:w257:errorcluster, 3:w258:refnum<k1>)  [unwired: 2 in, 1 out]
              n174 = Read Datalog(4:w257, 6:-1 ("count (1)"), 7:w258) -> (0:w262:errorcluster, 2:w243:T9, 3:w261:refnum<k1>)
              n175 = Close File(refnum=w261, error in=w262) -> (error out=→"error out 9":errorcluster)  [unwired: 1 out]
              n176 = case shown="False" w237 {
                tunnel: w244 -> [w288 _]
                tunnel: w243 -> [w287 _]
                tunnel: [w286 w332] -> w242
                tunnel: w240 -> [w285 _]
                tunnel: w239 -> [w284 w332]
                frame False {
                  n177 = for {
                    tunnel: w284 -> [w292]
                    tunnel: w288 -> [w303]
                    tunnel: w287 -> [w299] mode=indexing
                    tunnel: [w291] -> w286
                    tunnel: w285 -> [w289]
                    (unwired) timestamp(0 s since 1904-01-01) ("OUTPUT_DATE")
                    w297 = 0  # number copy to print
                    n178 = Unbundle By Name(w299) -> ("Invoice"=w301:string, "Item Code"=w300:string)
                    n179 = Bundle By Name(cluster=T11 {"Row"=0, "Column"=0} ("Index Values"), "Row"=0 ("index of element")) -> (w296:T11)
                    n180 = Increment(x=w297) -> ()  [unwired: 1 out]
                    n181 = property on="Table 2" class="Tbl (strict)"("Index Values"=w296) -> ()  [unwired: 2 in, 2 out]
                    n182 = Format Into String(format string="`%s`.`%s`", w303, w300) -> (resulting string=w293:string)  [unwired: 2 in, 1 out]
                    n183 = Format Into String(format string="`%s`.`STORE_INPUT_%s`", w303, w301) -> ()  [unwired: 2 in, 2 out]
                    n184 = for {
                      N: 1 -> [_]
                      tunnel: w299 -> [w324]
                      tunnel: w293 -> [w311]
                      shift-right: [w306] -> w291
                      shift-left: w292 -> [w310]
                      tunnel: w289 -> [w304]
                      stop <- w307 continue-if-true
                      (unwired) "" ("LOT_MAKER")
                      (unwired) "" ("OUTPUT_NO")
                      (unwired) T12 {"ITEM_CODE"="", "INVOICE_NO"="", "INVOICE_DATE"=timestamp(0 s since 1904-01-01), "LOT_MAKER"="", "QUANTITY"=0.0, "INVOICE_ECODE"="", "INPUT_NO"="", "INPUT_DATE"=timestamp(0 s since 1904-01-01), "INPUT_ECODE"="", "LINEBACK_NO"="", "LINEBACK_DATE"=timestamp(0 s since 1904-01-01), "LINEBACK_ECODE"="", "OUTPUT_NO"="", "OUTPUT_DATE"=timestamp(0 s since 1904-01-01), "OUTPUT_ECODE"="", "DESTINATION"=""}
                      n185 = Unbundle By Name(w324) -> ("Invoice"=w309:string, "Output Date"=w319:string, "Output No."=w316:string, "Input"=w313:string, "Worker Code"=w315:string)  [unwired: 2 out]
                      n186 = Wait (ms)(milliseconds to wait=w304) -> ()  [unwired: 1 out]
                      n187 = Scan From String(format string="%<%d-%b-%Y-%H-%M-%S>T", input string=w319, default 1=i64 0) -> (error out=→"error out 4":errorcluster, output 1=w321:i64)  [unwired: 2 in, 2 out]
                      n188 = To Time Stamp(1:w321) -> (0:w317:timestamp)
                      n189 = Format Into String(format string="WHERE INPUT_NO='%s' AND QUANTITY='%s' AND OUTPUT_NO='' LIMIT 1" ("condition"), w309, w313) -> (resulting string=w312:string)  [unwired: 2 in, 1 out]
                      n190 = Bundle(w317, "Output No."=w316, "Worker Code"=w315) -> (w314:T14)  [unwired: 1 in]
                      n191 = call <vilib>:"DB Tools Update Data.vi"("condition"=w312, "data"=w314, "columns"=string[] ["OUTPUT_DATE", "OUTPUT_NO", "OUTPUT_ECODE"], "table"=w311, "connection reference"=w310) -> ("error out"=w307:errorcluster, "connection reference out"=w305:T1)  [unwired: 5 in]
                      n192 = case shown="Error" w307 {
                        tunnel: [w325 w326] -> w306
                        tunnel: w305 -> [w325 _]
                        frame No Error {
                        }
                        frame Error {
                          n193 = disable-structure shown="Enabled" {
                            disable-tunnel: [w327 "connection reference 3"] -> _
                            disable-tunnel: [w327 _] -> w326
                            frame Enabled {
                              n194 = call-poly <vilib>:"DB Tools Open Connection.vi"("password"="871994" ("userID"), "userID"="hoangbao2106", "connection information"="Database" ("userID")) -> ("connection reference"=w327:T1)  [unwired: 5 in, 1 out]
                            }
                            frame Disabled {
                            }
                          }
                        }
                      }
                    }
                  }
                }
                frame True {
                }
              }
              n195 = call <vilib>:"DB Tools Close Connection.vi"("connection reference"=w242) -> ("error out"=w241:errorcluster)  [unwired: 6 in]
              n196 = case shown="No Error" w241 {
                selector: w241 -> [w338 _]
                tunnel: w239 -> [_ w340]
                tunnel: [w338 w339] -> w236
                frame No Error {
                }
                frame Error {
                  n197 = call <vilib>:"DB Tools Close Connection.vi"("connection reference"=w340) -> ("error out"=w339:errorcluster)  [unwired: 6 in]
                }
              }
              "Numeric" <- w238
            }
            "Array" <- w198
            n198 = Close File(refnum=w213, error in=w214) -> (path=w202:path, error out=→"error out 6":errorcluster)
            n199 = Index Array(array=w205, index=0) -> (element=w208:T3)
            n200 = call "Delete File Temp.vi"("Source Path"=w201, "Temp path"=w202) -> ()  [unwired: 8 in, 2 out]
            n201 = Unbundle By Name(w208) -> ("Initial"=w207:string)
            n202 = case shown="\"\"" w207 {
              selector: w207 -> [w229 _]
              tunnel: [w229 "29-Nov-2015-07-00-00"] -> w206
              frame Default {
              }
              frame "" {
              }
            }
            n203 = local write "Initial Date"(w206) -> ()
          }
        }
      }
      event "End": Value Change {
        n204 = event-data() -> ()  [unwired: 1 in, 6 out]
        n205 = Build Path(base path="Data\\", name or relative path="Password.dat") -> (appended path=w446:path)
        n206 = call "Open File Temp.vi"("Path file"=w446) -> ("Source Path"=w443:path, "Temp path"=w445:path)  [unwired: 7 in, 2 out]
        n207 = Open/Create/Replace Datalog(5:"output cluster 2", 9:enum16{"read/write", "read-only", "write-only"}."read/write" ("access (0:read/write)"), 10:T8."open or create" ("operation (0:open)"), 11:w445) -> (0:w449:errorcluster, 3:w450:refnum<k1>)  [unwired: 2 in, 1 out]
        n208 = Read Datalog(4:w449, 6:-1 ("count (1)"), 7:w450) -> (0:w447:errorcluster, 2:w442:cluster{"ID":string, "Password":string}[], 3:w448:refnum<k1>)
        "password" <- w442
        n209 = local read "Ring"() -> (w457:u16)
        n210 = case shown="1" w457 {
          tunnel: w442 -> [w458 w501]
          frame 1 {
            n211 = Index Array(array=w458, index=0) -> (element=w459:cluster{"ID":string, "Password":string})
            n212 = call "PASS.vi"() -> ("Password"=w465:string, "ID"=w467:string)  [unwired: 16 in, 2 out]
            n213 = Unbundle By Name(w459) -> ("ID"=w466:string, "Password"=w464:string)
            n214 = Equal?(x=w467, y=w466) -> (x = y?=w463:bool)
            n215 = Equal?(x=w465, y=w464) -> (x = y?=w462:bool)
            n216 = And(x=w463, y=w462) -> (x .and. y?=w461:bool)
            n217 = case shown="True" w461 {
              frame False {
                n218 = call "Display Message to User4"() -> ()  [unwired: 10 in, 2 out]
              }
              frame True {
                n219 = call "Display Message to User"() -> ("OK"=w468:bool)  [unwired: 10 in, 1 out]
                n220 = case shown="True" w468 {
                  frame False {
                  }
                  frame True {
                    n221 = call "Display Message to User2"() -> ("OK"=w469:bool)  [unwired: 10 in, 1 out]
                    n222 = case shown="True" w469 {
                      frame False {
                      }
                      frame True {
                        w472 = TRUE ("Message")
                        n223 = local read "PRODUCT"() -> (w480:string)
                        n224 = local read "Table"() -> (w482:string[][])
                        n225 = for {
                          tunnel: w482 -> [w500] mode=indexing
                          tunnel: [w493] -> w487 mode=indexing
                          w496 = T15 {"Item Code"="", "Initial"="", "Stock"=""}  # end
                          n226 = Index Array(array=w500, index #1=2 ("index"), index #2=9 ("index")) -> (element #1=w497:string, element #2=w494:string)
                          n227 = local read "DATE"() -> (w495:string)
                          n228 = Bundle By Name(cluster=w496, "Item Code"=w497, "Stock"=w494, "Initial"=w495) -> (w493:T15)
                        }
                        n229 = Concatenate Strings(w480, "\\" ("string"), "linestock.dat" ("name or relative path")) -> (w477:string)
                        n230 = local read "Data\\"() -> (w483:path)
                        n231 = Build Path(base path=w483, name or relative path=w477) -> (appended path=w476:path)
                        n232 = local read "element"() -> (w481:T3)
                        n233 = call "Open File Temp.vi"("Write?"=w472, "Path file"=w476) -> ("Deny File Refnum"=w471:refnum<k1>, "Source Path"=w473:path, "Temp path"=w475:path)  [unwired: 6 in, 1 out]
                        n234 = Open/Create/Replace Datalog(5:w481, 9:enum16{"read/write", "read-only", "write-only"}."read/write" ("access (0:read/write)"), 10:T8."replace or create" ("operation (0:open)"), 11:w475) -> (0:w488:errorcluster, 3:w486:refnum<k1>)  [unwired: 2 in, 1 out]
                        n235 = Write Datalog(4:w488, 6:w487, 7:w486) -> (0:w490:errorcluster, 3:w489:refnum<k1>)
                        n236 = Close File(refnum=w489, error in=w490) -> (path=w474:path, error out=w470:errorcluster)
                        n237 = case shown="No Error" w470 {
                          frame No Error {
                            n238 = property on="End" class="Bool"("Visible"=FALSE) -> ()  [unwired: 2 in, 2 out]
                            n239 = property on="End" class="Bool"("DisabledEnum"=T6."Disabled" ("Disabled")) -> ()  [unwired: 2 in, 2 out]
                          }
                          frame Error {
                          }
                        }
                        n240 = call "Delete File Temp.vi"("Deny File Refnum"=w471, "Source Path"=w473, "Write?"=w472, "Temp path"=w474) -> ()  [unwired: 6 in, 2 out]
                      }
                    }
                  }
                }
              }
            }
          }
          frame 0, Default {
            n241 = Index Array(array=w501, index=0) -> (element=w502:cluster{"ID":string, "Password":string})
            n242 = call "PASS.vi"() -> ("Password"=w508:string, "ID"=w510:string)  [unwired: 16 in, 2 out]
            n243 = Unbundle By Name(w502) -> ("ID"=w509:string, "Password"=w507:string)
            n244 = Equal?(x=w510, y=w509) -> (x = y?=w506:bool)
            n245 = Equal?(x=w508, y=w507) -> (x = y?=w505:bool)
            n246 = And(x=w506, y=w505) -> (x .and. y?=w504:bool)
            n247 = case shown="True" w504 {
              frame False {
                n248 = call "Display Message to User3"() -> ()  [unwired: 10 in, 2 out]
              }
              frame True {
                n249 = call "Display Message to User5"() -> ("OK"=w511:bool)  [unwired: 10 in, 1 out]
                n250 = case shown="True" w511 {
                  frame False {
                  }
                  frame True {
                    n251 = call "Display Message to User6"() -> ("OK"=w512:bool)  [unwired: 10 in, 1 out]
                    n252 = case shown="True" w512 {
                      frame False {
                      }
                      frame True {
                        w514 = TRUE ("Message")
                        n253 = local read "PRODUCT"() -> (w522:string)
                        n254 = local read "Table"() -> (w524:string[][])
                        n255 = for {
                          tunnel: w524 -> [w540] mode=indexing
                          tunnel: [w533] -> w529 mode=indexing
                          w536 = T15 {"Item Code"="", "Initial"="", "Stock"=""}  # end
                          n256 = Index Array(array=w540, index #1=2 ("index"), index #2=9 ("index")) -> (element #1=w537:string, element #2=w534:string)
                          n257 = local read "DATE"() -> (w535:string)
                          n258 = Bundle By Name(cluster=w536, "Item Code"=w537, "Stock"=w534, "Initial"=w535) -> (w533:T15)
                        }
                        n259 = Concatenate Strings(w522, "\\" ("string"), "invoicestock.dat" ("name or relative path")) -> (w519:string)
                        n260 = local read "Data\\"() -> (w525:path)
                        n261 = Build Path(base path=w525, name or relative path=w519) -> (appended path=w518:path)
                        n262 = local read "element"() -> (w523:T3)
                        n263 = call "Open File Temp.vi"("Write?"=w514, "Path file"=w518) -> ("Deny File Refnum"=w513:refnum<k1>, "Source Path"=w515:path, "Temp path"=w517:path)  [unwired: 6 in, 1 out]
                        n264 = Open/Create/Replace Datalog(5:w523, 9:enum16{"read/write", "read-only", "write-only"}."read/write" ("access (0:read/write)"), 10:T8."replace or create" ("operation (0:open)"), 11:w517) -> (0:w530:errorcluster, 3:w528:refnum<k1>)  [unwired: 2 in, 1 out]
                        n265 = Write Datalog(4:w530, 6:w529, 7:w528) -> (0:w532:errorcluster, 3:w531:refnum<k1>)
                        n266 = Close File(refnum=w531, error in=w532) -> (path=w516:path)  [unwired: 1 out]
                        n267 = call "Delete File Temp.vi"("Deny File Refnum"=w513, "Source Path"=w515, "Write?"=w514, "Temp path"=w516) -> ()  [unwired: 6 in, 2 out]
                      }
                    }
                  }
                }
              }
            }
          }
        }
        n268 = Close File(refnum=w448, error in=w447) -> (path=w444:path)  [unwired: 1 out]
        n269 = call "Delete File Temp.vi"("Source Path"=w443, "Temp path"=w444) -> ()  [unwired: 8 in, 2 out]
      }
      event "Find": Value Change {
        n270 = event-data() -> ("NewVal"=w541:string)  [unwired: 1 in, 5 out]
        n271 = local read "Table"() -> (w542:string[][])
        n272 = Index Array(array=w542, index (col)=2 ("disabled index (col)")) -> (element=w544:string[])  [unwired: 1 in]
        n273 = for {
          tunnel: w544 -> [w556] mode=indexing
          tunnel: w541 -> [w555]
          shift-right: [w553] -> w547
          shift-left: i32[] [] ("Find Array") -> [w552]
          shift-right: [w549] -> _
          shift-left: 0 -> [w550]
          i -> [w551]
          n274 = Search and Replace String(input string=w556, search string=w555, replace string=w555) -> (number of replacements=w554:i32)  [unwired: 5 in, 3 out]
          n275 = case shown="0" w554 {
            tunnel: [w558 w561] -> w553
            tunnel: w552 -> [w558 w563]
            tunnel: w551 -> [_ w562]
            tunnel: w550 -> [w557 w560]
            tunnel: [w557 w559] -> w549
            frame 0 {
            }
            frame 1, Default {
              n276 = Increment(x=w560) -> (x+1=w559:i32)
              n277 = Insert Into Array(array=w563, index=w560, new element=w562) -> (w561:i32[])
            }
          }
        }
        n278 = local write "Find Array"(w547) -> ()
        n279 = Empty Array?(array=w547) -> (empty?=w548:bool)
        n280 = case shown="True" w548 {
          tunnel: w541 -> [_ w569]
          tunnel: w547 -> [w566 _]
          frame False {
            n281 = Index Array(array=w566, index=0) -> (element=w564:i32)
            n282 = Bundle By Name(cluster=T11 {"Row"=0, "Column"=0} ("Index Values"), "Row"=w564) -> (w568:T11)
            n283 = property on="Table" class="Tbl (strict)"("Index Values"=w568) -> ()  [unwired: 2 in, 2 out]
          }
          frame True {
            n284 = local read "Table"() -> (w575:string[][])
            n285 = Index Array(array=w575, index (col)=3 ("disabled index (col)")) -> (element=w572:string[])  [unwired: 1 in]
            n286 = for {
              tunnel: w572 -> [w584] mode=indexing
              tunnel: w569 -> [w583]
              shift-right: [w581] -> w570
              shift-left: i32[] [] ("Find Array") -> [w580]
              shift-right: [w577] -> _
              shift-left: 0 -> [w578]
              i -> [w579]
              n287 = Search and Replace String(input string=w584, search string=w583, replace string=w583) -> (number of replacements=w582:i32)  [unwired: 5 in, 3 out]
              n288 = case shown="1, Default" w582 {
                tunnel: [w586 w589] -> w581
                tunnel: w580 -> [w586 w591]
                tunnel: w579 -> [_ w590]
                tunnel: w578 -> [w585 w588]
                tunnel: [w585 w587] -> w577
                frame 0 {
                }
                frame 1, Default {
                  n289 = Increment(x=w588) -> (x+1=w587:i32)
                  n290 = Insert Into Array(array=w591, index=w588, new element=w590) -> (w589:i32[])
                }
              }
            }
            n291 = local write "Find Array"(w570) -> ()
            n292 = Empty Array?(array=w570) -> (empty?=w571:bool)
            n293 = case shown="False" w571 {
              tunnel: w570 -> [w594 _]
              frame False {
                n294 = Index Array(array=w594, index=0) -> (element=w593:i32)
                n295 = Bundle By Name(cluster=T11 {"Row"=0, "Column"=0} ("Index Values"), "Row"=w593) -> (w592:T11)
                n296 = property on="Table" class="Tbl (strict)"("Index Values"=w592) -> ()  [unwired: 2 in, 2 out]
              }
              frame True {
              }
            }
          }
        }
      }
      event "Exit": Value Change {
        n297 = event-data() -> ()  [unwired: 1 in, 6 out]
      }
    }
  }
  n298 = call "Open File Temp.vi"("Path file"=w8) -> ("Source Path"=w5:path, "Temp path"=w7:path)  [unwired: 7 in, 2 out]
  n299 = Format Date/Time String(time format string (%c)="%d-%b-%Y-%H-%M-%S", seconds (now)=w20) -> (date/time string=w11:string)  [unwired: 1 in]
  n300 = Open/Create/Replace Datalog(5:w16, 11:w7) -> (0:w18:errorcluster, 3:w17:refnum<k1>)  [unwired: 4 in, 1 out]
  n301 = local write "DATE"(w11) -> ()
  n302 = Read Datalog(4:w18, 6:-1 ("count (1)"), 7:w17) -> (0:w12:errorcluster, 2:w10:T4, 3:w13:refnum<k1>)
  "Item data" <- w10
  n303 = for {
    tunnel: w10 -> [w603] mode=indexing
    shift-right: [w601] -> w1
    shift-left: string[] [] -> [w600]
    i -> [w598]
    n304 = Unbundle By Name(w603) -> ("Item Code"=w599:string)
    n305 = Search 1D Array(1D array=w600, element=w599) -> (index of element=w602:i32)  [unwired: 1 in]
    n306 = case shown="-1" w602 {
      tunnel: [w604 w606] -> w601
      tunnel: w600 -> [w604 w608]
      tunnel: w599 -> [_ w607]
      frame 0, Default {
      }
      frame -1 {
        n307 = Insert Into Array(array=w608, index=0, new element=w607) -> (w606:string[])
      }
    }
    "Numeric 2" <- w598
  }
  "Item code" <- w1
  n308 = Close File(refnum=w13, error in=w12) -> (path=w6:path)  [unwired: 1 out]
  n309 = call "Delete File Temp.vi"("Source Path"=w5, "Temp path"=w6) -> ()  [unwired: 8 in, 2 out]
